vi "VI Server_Open VI Controls Refs_LabelsFromVI Reference.vi"(8 "error in (no error)":errorcluster, 11 "Target VI Ref.":refnum<vi>) -> (0 "error out":errorcluster, 3 "VI Server Cluster.OUT":T1)   [LabVIEW 2020, in "VI Server Toolkit LV2013.lvlib"]
doc: "Generates VI Server Cluster from targeted VI reference.\nUsually used in conjunction with Static VI reference."
uses:
  VI Server Toolkit LV2013.lvlib
  VI Server_TypeDefs/VI Server_RefsCluster.ctl
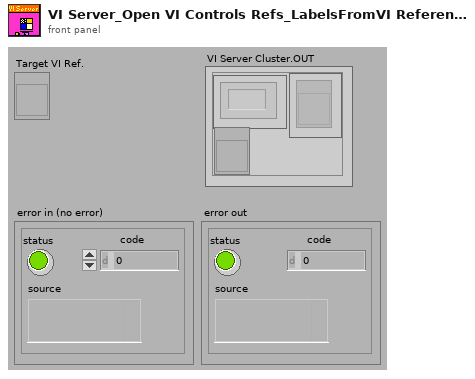
[diagram p1: front panel]
types:
  T1 = typedef "VI Server_RefsCluster.ctl" = cluster{"Labels":string[], "Refs":refnum<vi>[], "VI Ref":refnum<vi>}
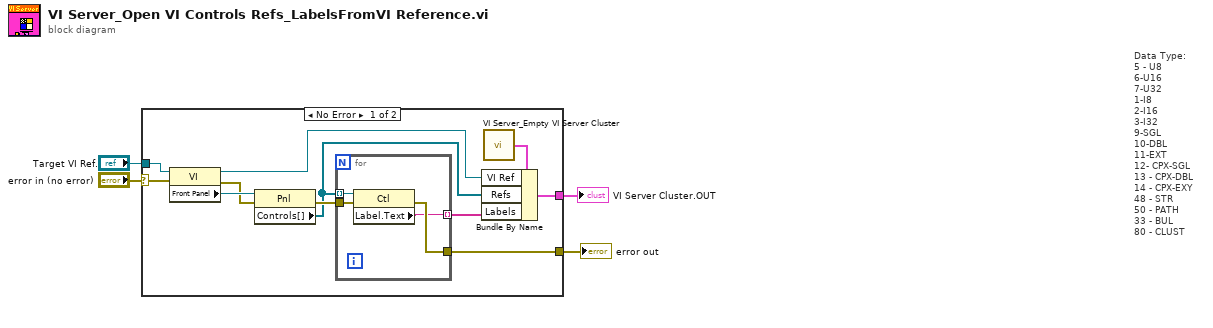
[diagram p0: block diagram]
diagram:
  # "Data Type:\n5 - U8\n6-U16\n7-U32\n1-I8\n2-I16\n3-I32\n9-SGL\n10-DBL\n11-EXT\n12- CPX-SGL\n13 - CPX-DBL\n14 - CPX-EXY\n48 - STR\n50 - PATH\n33 - BUL\n80 - CLUST"
  n1 = case shown="No Error" "error in (no error)" {
    selector: "error in (no error)" -> [w6 w20]
    tunnel: [w12 w20] -> w4
    tunnel: [w11 _] -> w3
    tunnel: "Target VI Ref." -> [w7 _]
    frame No Error {
      n2 = property class="VI"(reference=w7, error in=w6) -> (reference out=w9:refnum<vi>, error out=w14:errorcluster, "Front Panel"=w15:refnum<vi>)
      n3 = property class="Pnl"(reference=w15, error in=w14) -> (error out=w13:errorcluster, "Controls[]"=w8:refnum<vi>[])  [unwired: 1 out]
      n4 = for {
        tunnel: w8 -> [w19] mode=indexing
        tunnel: w13 -> [w18]
        tunnel: [w17] -> w12
        tunnel: [w16] -> w10 mode=indexing
        n5 = property class="Ctl"(reference=w19, error in=w18) -> (error out=w17:errorcluster, "Label.Text"=w16:string)  [unwired: 1 out]
      }
      n6 = call "VI Server_Empty VI Server Cluster.vi"() -> ("VI Server Cluster"=w5:T1)  [unwired: 7 in]
      n7 = Bundle By Name(cluster=w5, "VI Ref"=w9, "Refs"=w8, "Labels"=w10) -> (w11:T1)
    }
    frame Error {
    }
  }
  "error out" <- w4
  "VI Server Cluster.OUT" <- w3
